vi "run.end.vi"(8 "error in":errorcluster, 11 "Run in":refnum<class "Run.lvclass">) -> (0 "error out":errorcluster, 3 "Run out":refnum<class "Run.lvclass">)   [LabVIEW 2020, in "Run.lvclass"]
doc: "Returns the run's end time and whether one has been set."
uses:
  Run.lvclass
  Run.lvclass/Run.ctl
  client.lvlib
panel:
  out "out_millis out":dbl
  out "is_present out":bool
  in  "out_millis":dbl
  in  "is_present":bool
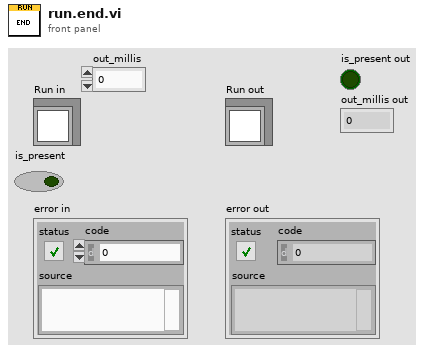
[diagram p1: front panel]
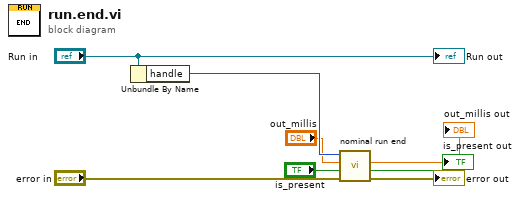
[diagram p0: block diagram]
diagram:
  n1 = Unbundle By Name("Run in") -> ("handle"=w6:i32)
  n2 = call "nominal run end.vi"("error in (no error)"="error in", "is_present"="is_present", "out_millis"="out_millis", "run"=w6) -> ("error out"=→"error out":errorcluster, "is_present out"=→"is_present out":bool, "out_millis out"=→"out_millis out":dbl)  [unwired: 4 in, 1 out]
  "Run out" <- "Run in"
